vi "Get Debug DLL Path.vi"() -> (0 "DLL Path":path)   [LabVIEW 2019, in "grpc-lvsupport.lvlib"]
uses:
  grpc-lvsupport.lvlib
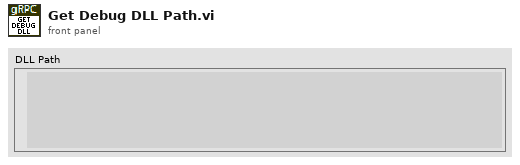
[diagram p1: front panel]
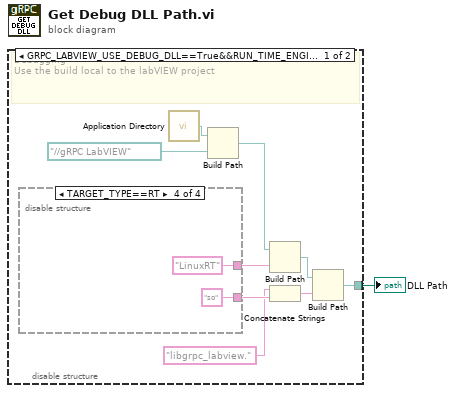
[diagram p0: block diagram]
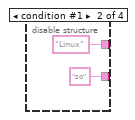
[diagram p3: hidden frame]
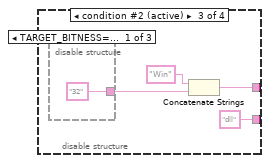
[diagram p4: hidden frame]
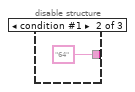
[diagram p5: hidden frame]
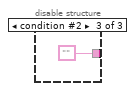
[diagram p6: hidden frame]
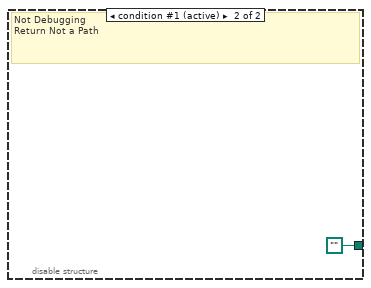
[diagram p7: hidden frame]
diagram:
  n1 = disable-structure shown="GRPC_LABVIEW_USE_DEBUG_DLL==True&&RUN_TIME_ENGINE==False" {
    disable-tunnel: [w3 path ""] -> w1
    frame condition #0 {
      # "Debugging\nUse the build local to the labVIEW project"
      n2 = disable-structure shown="TARGET_TYPE==RT" {
        disable-tunnel: [_ "so" "dll" "so"] -> w7
        disable-tunnel: [_ "Linux" w14 "LinuxRT"] -> w4
        frame condition #0 {
        }
        frame condition #1 {
        }
        frame condition #2 (active) {
          n3 = disable-structure shown="TARGET_BITNESS==32" {
            disable-tunnel: ["32" "64" ""] -> w15
            frame condition #0 (active) {
            }
            frame condition #1 {
            }
            frame condition #2 {
            }
          }
          n4 = Concatenate Strings("Win" ("string"), w15) -> (w14:string)
        }
        frame condition #3 {
        }
      }
      n5 = call <vilib>:"Application Directory.vi"() -> ("Application Directory"=w8:path)
      n6 = Build Path(base path=w8, name or relative path=path "../../gRPC LabVIEW") -> (appended path=w9:path)
      n7 = Build Path(base path=w9, name or relative path=w4) -> (appended path=w10:path)
      n8 = Concatenate Strings("libgrpc_labview." ("format string"), w7) -> (w2:string)
      n9 = Build Path(base path=w10, name or relative path=w2) -> (appended path=w3:path)
    }
    frame condition #1 (active) {
      # "Not Debugging\nReturn Not a Path"
    }
  }
  "DLL Path" <- w1
